vi "UpdateGraphs.vi"(8 "error in (no error)":errorcluster, 10 "Channels in":string[](array[string]), 11 ".NET Refnum in":T1) -> (0 "error out":errorcluster, 2 "Array":waveform(dbl)[](array[waveform]), 3 ".NET Refnum out":T1)   [LabVIEW 2017]
uses:
  <vilib>/NI Veristand/Execution/Workspace/WorkspaceAPI.ctl
  NationalInstruments.VeriStand.ClientAPI
  <vilib>/NI Veristand/Execution/Workspace/NI VeriStand - Get Multiple Channel Values.vi
  <vilib>/NI Veristand/Execution/Workspace/NI_VS Workspace ExecutionAPI.lvlib
panel:
  in  "dt (s)":dbl=100.0 format="%#_13g"
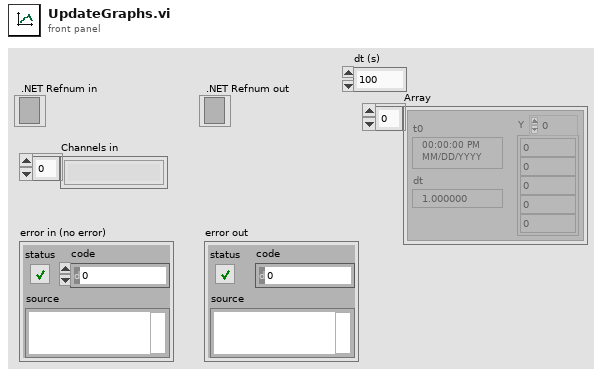
[diagram p1: front panel]
types:
  T1 = typedef "NI_VS Workspace ExecutionAPI.lvlib/WorkspaceAPI.ctl" = refnum<k24>
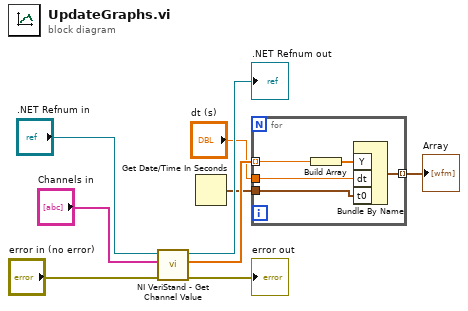
[diagram p0: block diagram]
diagram:
  n1 = call-poly <vilib>:"NI VeriStand - Get Channel Value.vi"("error in (no error)"="error in (no error)", "Channels"="Channels in", "WorkspaceManager in"=".NET Refnum in") -> ("error out"=→"error out":errorcluster, "Values"=w4:dbl[], "WorkspaceManager out"=→".NET Refnum out":T1)  [unwired: 6 in]
  n2 = Get Date/Time In Seconds() -> (seconds since 1Jan1904=w3:timestamp)
  n3 = for {
    tunnel: w4 -> [w11] mode=indexing
    tunnel: w3 -> [w13]
    tunnel: "dt (s)" -> [w12]
    tunnel: [w10] -> w1 mode=indexing
    n4 = Build Array(w11) -> (w14:dbl[])
    n5 = Bundle By Name("Y"=w14, "dt"=w12, "t0"=w13) -> (w10:waveform(dbl))  [unwired: 1 in]
  }
  "Array" <- w1
